vi "Write Attribue Tree.vi"() -> ()   [LabVIEW 2014]
panel:
  in  "Tree":string(tree)
  in  "Array":string[][](array[string])
  out "Suceed updating?":bool
  out "Updated Value":string
  in  "Value":string
  in  "Active Item:Tag":string
  out "All Tags":string[](array[string])
  in  "Attribute Tree":string(tree)
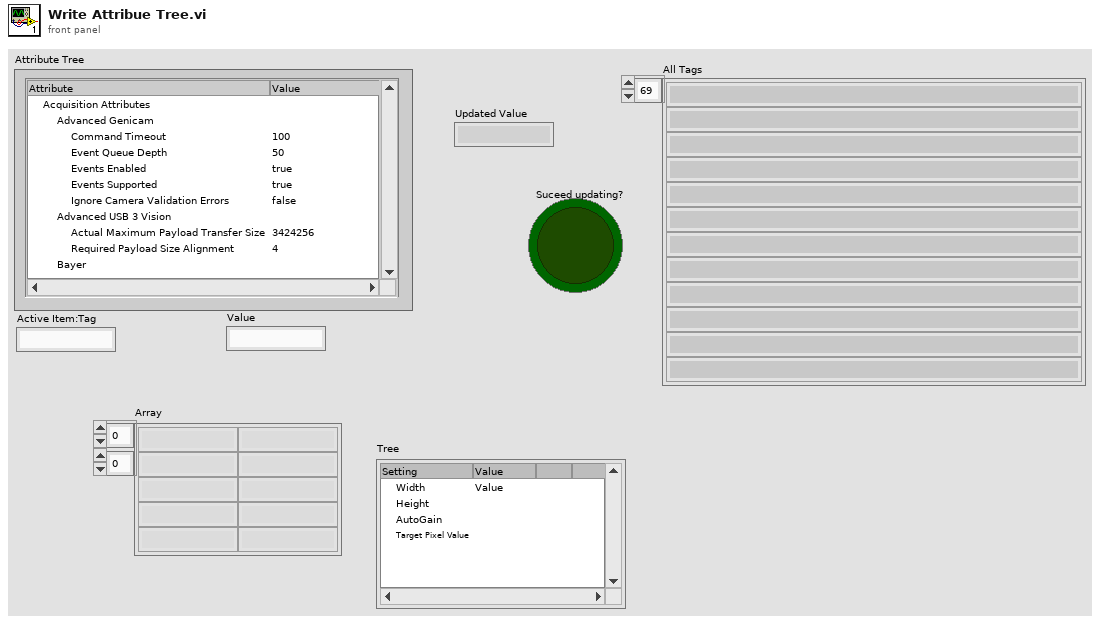
[diagram p1: front panel]
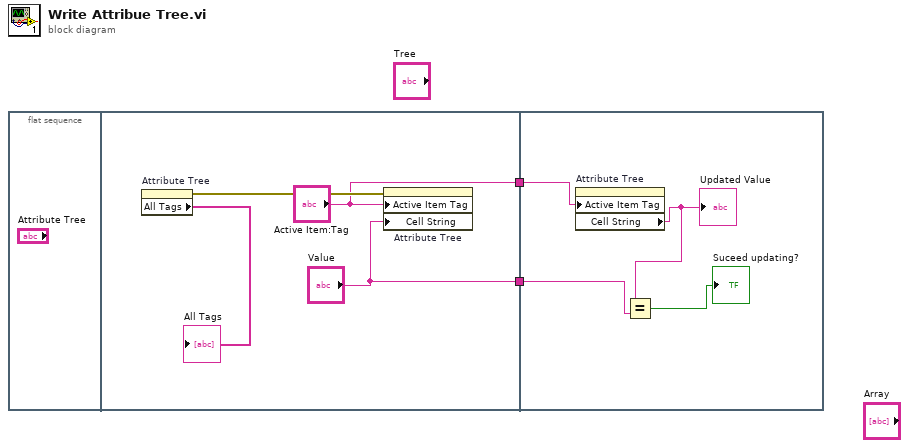
[diagram p0: block diagram]
diagram:
  n1 = flat-sequence {
    tunnel: ["Active Item:Tag"] -> w2
    tunnel: ["Value"] -> w1
    tunnel: w2 -> [w10]
    tunnel: w1 -> [w9]
    frame #0 {
    }
    frame #1 {
      n2 = property on="Attribute Tree" class="Tree (strict)"() -> (error out=w5:errorcluster, "All Tags"=→"All Tags":string[])  [unwired: 2 in, 1 out]
      n3 = property on="Attribute Tree" class="Tree (strict)"(error in=w5, "Active Item Tag"="Active Item:Tag", "Cell String"="Value") -> ()  [unwired: 1 in, 2 out]
    }
    frame #2 {
      n4 = property on="Attribute Tree" class="Tree (strict)"("Active Item Tag"=w10) -> ("Cell String"=w8:string)  [unwired: 2 in, 2 out]
      "Updated Value" <- w8
      n5 = Equal?(x=w8, y=w9) -> (x = y?=→"Suceed updating?":bool)
    }
  }
